vi "Set Mask.vi"(7 "Mask":bool[](array[boolean])=[FALSE, FALSE, FALSE, FALSE, FALSE, FALSE, FALSE, FALSE], 8 "error in (no error)":errorcluster, 10 "Address (0)":i32, 11 "VISA resource name":refnum<visa-resource-name>) -> (0 "error out":errorcluster, 3 "VISA resource name out":refnum<visa-resource-name>)   [LabVIEW 2021, in "Environment Chamber.lvlib" / "Climatic Chamber.lvlib"]
doc: "<b>Interrupt mask setting</B>\n\nPerforms the mask setting of the SRQ (Service Request) status.\n\nSRQ1: Not used\nSRQ2: When an alarm occurs on the chamber, 1 is set.\nSRQ3: When a single-step operation ends in remote program mode, 1 is set.\nSRQ4: When the state transitions from power off to operation, or vice versa, 1 isset.\nSRQ5: Not used\nSRQ6: Not used\nSRQ7: Reserved with the SRQ function for GPIB communication\nSRQ8: Not used"
uses:
  Climatic Chamber.lvlib
panel:
  out "NACK":bool
  out "Error":bool
  out "ACK":bool
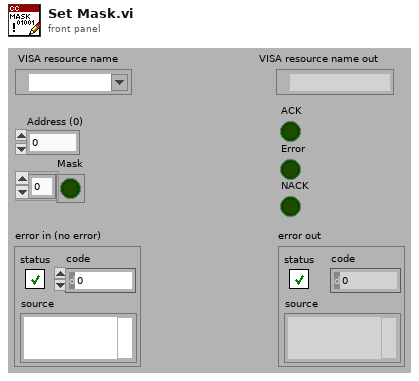
[diagram p1: front panel]
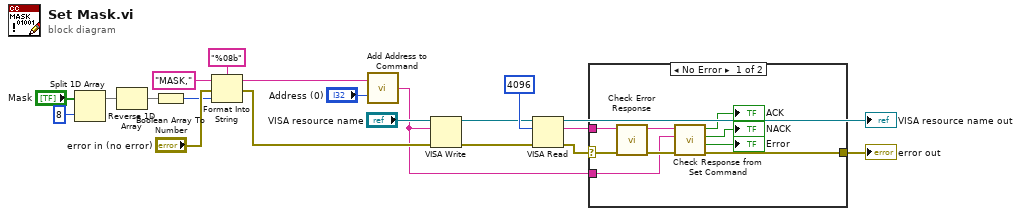
[diagram p0: block diagram]
diagram:
  n1 = Split 1D Array(array="Mask", index=8) -> (first subarray=w4:bool[])  [unwired: 1 out]
  n2 = Reverse 1D Array(array=w4) -> (reversed array=w1:bool[])
  n3 = Boolean Array To Number(Boolean array=w1) -> (number=w3:u32)
  n4 = Format Into String(format string="%08b", initial string="MASK,", error in="error in (no error)", w3) -> (resulting string=w8:string, error out=w7:errorcluster)
  n5 = call "Add Address to Command.vi"("Address (0)"="Address (0)", "Command"=w8) -> ("Command OUT"=w6:string)
  n6 = VISA Write(VISA resource name="VISA resource name", write buffer=w6, error in (no error)=w7) -> (VISA resource name out=w17:refnum<visa-resource-name>, error out=w16:errorcluster)  [unwired: 1 out]
  n7 = VISA Read(VISA resource name=w17, byte count=u32 4096, error in (no error)=w16) -> (VISA resource name out=→"VISA resource name out":refnum<visa-resource-name>, read buffer=w12:string, error out=w13:errorcluster)  [unwired: 1 out]
  n8 = case shown="No Error" w13 {
    selector: w13 -> [w28 w30]
    tunnel: w12 -> [w29 _]
    tunnel: [w24 w30] -> w11
    tunnel: w6 -> [w25 _]
    frame No Error {
      n9 = call "Check Error Response.vi"("error in (no error)"=w28, "read String"=w29) -> ("error out"=w27:errorcluster, "String out"=w26:string)  [unwired: 7 in, 1 out]
      n10 = call "Check Response from Set Command.vi"("error in (no error)"=w27, "Command"=w25, "Response"=w26) -> ("error out"=w24:errorcluster, "Error"=→"Error":bool, "NACK"=→"NACK":bool, "ACK"=→"ACK":bool)  [unwired: 5 in]
    }
    frame Error {
    }
  }
  "error out" <- w11
